vi "1.dé_electronique_Led_Boucle.vi"() -> ()   [LabVIEW 2018]
panel:
  out "7":bool
  out "3":bool
  out "2":bool
  out "6":bool
  out "4":bool
  out "1":bool
  out "5":bool
  in  "Choisir le nbr":dbl
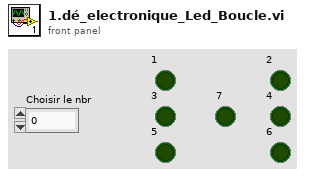
[diagram p1: front panel]
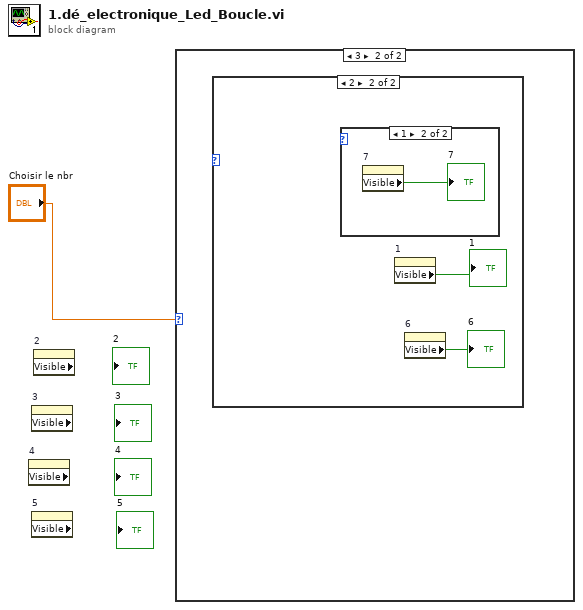
[diagram p0: block diagram]
diagram:
  n1 = property on="4" class="Bool (strict)" props=["Visible"]() -> ()  [unwired: 2 in, 3 out]
  n2 = property on="3" class="Bool (strict)" props=["Visible"]() -> ()  [unwired: 2 in, 3 out]
  n3 = property on="5" class="Bool (strict)" props=["Visible"]() -> ()  [unwired: 2 in, 3 out]
  n4 = property on="2" class="Bool (strict)" props=["Visible"]() -> ()  [unwired: 2 in, 3 out]
  n5 = case shown="3" "Choisir le nbr" {
    frame 0, Default {
    }
    frame 3 {
      n6 = case shown="2" {
        selector: _ -> [_ _]
        frame 0, Default {
        }
        frame 2 {
          n7 = case shown="1" {
            selector: _ -> [_ _]
            frame 0, Default {
            }
            frame 1 {
              n8 = property on="7" class="Bool (strict)"() -> ("Visible"=→"7":bool)  [unwired: 2 in, 2 out]
            }
          }
          n9 = property on="1" class="Bool (strict)"() -> ("Visible"=→"1":bool)  [unwired: 2 in, 2 out]
          n10 = property on="6" class="Bool (strict)"() -> ("Visible"=→"6":bool)  [unwired: 2 in, 2 out]
        }
      }
    }
  }
